vi "Take a Reading.vi"() -> ()   [LabVIEW 2018]
uses:
  EPU452 Class/EPU452.lvclass
panel:
  out "Readings":dbl[](array[numeric])=[0.0, 0.12, 0.0, 0.0]
  out "Units":string[](array[string])=["mS", "mS", "mS", "mS"]
  in  "COM Port":refnum<visa-resource-name>="COM3"
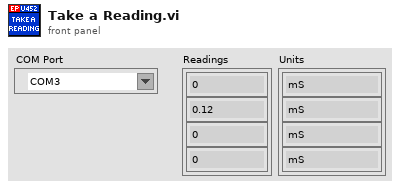
[diagram p1: front panel]
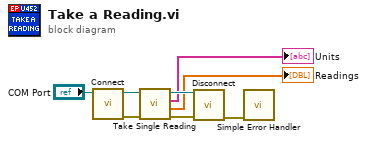
[diagram p0: block diagram]
diagram:
  n1 = call "Connect.vi"("COM Port"="COM Port") -> ("error out"=w5:errorcluster, "EPU452 out"=w6:refnum<class "EPU452.lvclass">)  [unwired: 9 in]
  n2 = call "Take Single Reading.vi"("error in (no error)"=w5, "EPU452 in"=w6) -> ("error out"=w4:errorcluster, "Readings"=→"Readings":dbl[], "Units"=→"Units":string[], "EPU452 out"=w7:refnum<class "EPU452.lvclass">)  [unwired: 5 in, 1 out]
  n3 = call "Disconnect.vi"("error in (no error)"=w4, "EPU452 in"=w7) -> ("error out"=w3:errorcluster)  [unwired: 9 in]
  n4 = call <vilib>:"Simple Error Handler.vi"("error in (no error)"=w3) -> ()  [unwired: 4 in, 5 out]
